vi "Visit.vi"(9 "Distance":u64, 10 "Position":cluster{i32, i32}, 11 "Map in":T1(c390)) -> (3 "Map out":T1(c390))   [LabVIEW 2023, in "d10.lvlib"]
uses:
  d10.lvlib
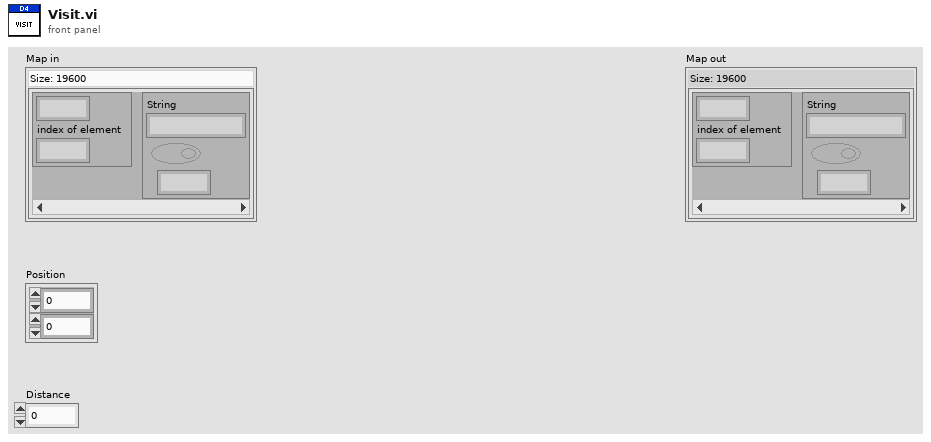
[diagram p1: front panel]
types:
  T1 = map{cluster{i32, "index of element":i32}, cluster{"String":string, bool, u64}}
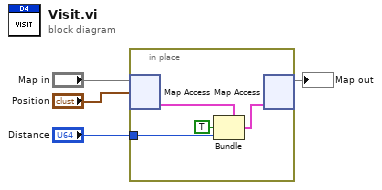
[diagram p0: block diagram]
diagram:
  n1 = in-place {
    in-place-border: "Distance" -> [w5]
    n2 = in-place-map #1("Map in", "Position") -> (w6:cluster{"String":string, bool, u64})  [unwired: 1 in, 1 out]
    n3 = Bundle(cluster=w6, TRUE, w5) -> (w7:cluster{"String":string, bool, u64})  [unwired: 1 in]
    n4 = in-place-map #1(w7) -> (→"Map out":T1)  [unwired: 1 in, 2 out]
  }
